vi "PMT communication_MD.vi"   [LabVIEW 2012]
uses:
  GFG/GFGstringGet.vi
  <vilib>/Instr/_visa.llb/VISA Configure Serial Port (Instr).vi
  GFG/GFGnumericGet.vi
  GFG/GFG library.lvlib
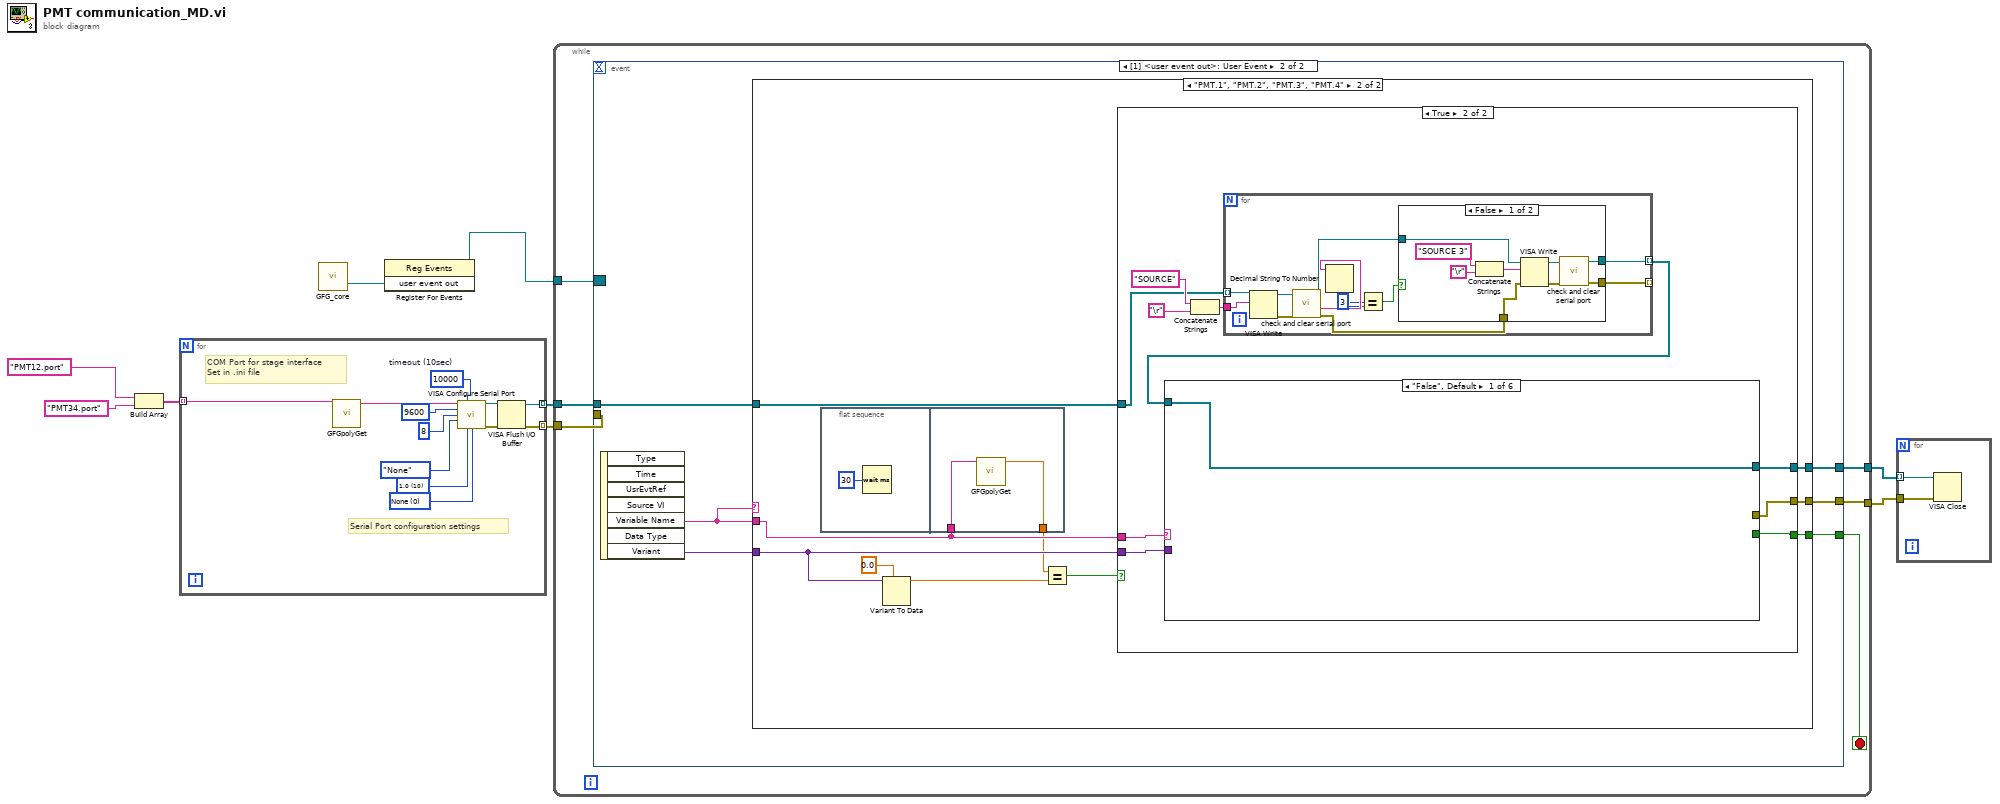
[diagram p0: block diagram]
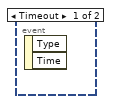
[diagram p2: hidden frame]
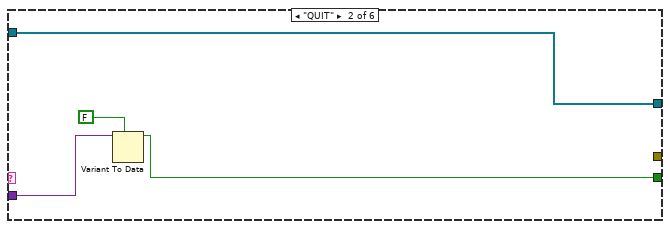
[diagram p6: hidden frame]
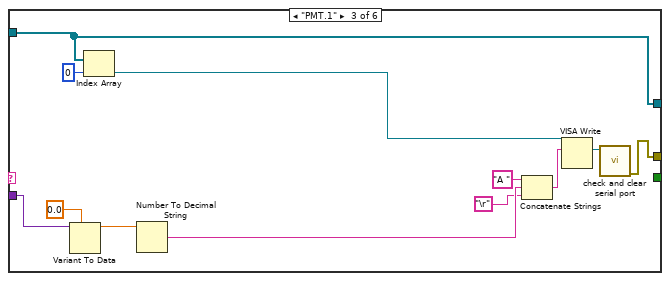
[diagram p7: hidden frame]
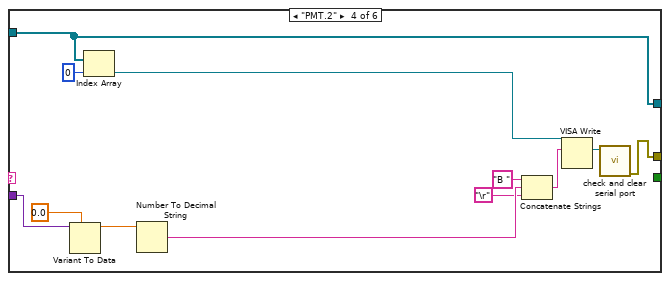
[diagram p8: hidden frame]
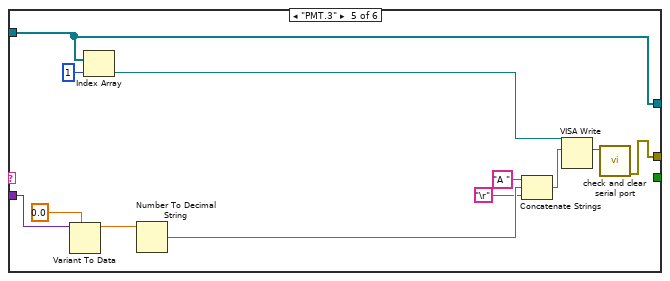
[diagram p9: hidden frame]
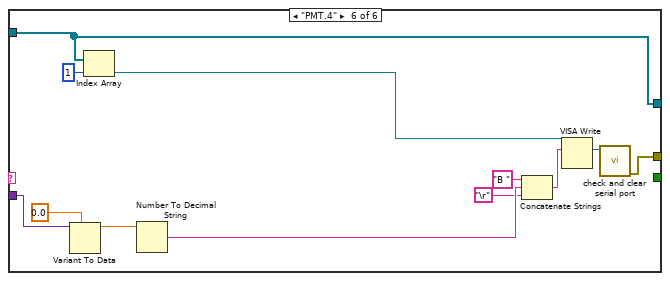
[diagram p10: hidden frame]
diagram:
  n1 = Build Array("PMT12.port" ("Variable Name in"), "PMT34.port" ("Variable Name in")) -> (w1:string[])
  n2 = for {
    tunnel: [w12] -> w9 mode=indexing
    tunnel: [w11] -> w8 mode=indexing
    tunnel: w1 -> [w10] mode=indexing
    w16 = u16 0 items=["None", "XON/XOFF", "RTS/CTS", "XON/XOFF & RTS/CTS", "DTR/DSR", "XON/XOFF & DTR/DSR"] ("flow control (0:none)")
    w17 = u16 10 items=["1.0"=10, "1.5"=15, "2.0"=20] ("stop bits (10: 1 bit)")
    w21 = u32 10000  # timeout (10sec)
    # "COM Port for stage interface\nSet in .ini file"
    # "Serial Port configuration settings"
    n3 = call-poly "GFGpolyGet.vi"("Variable Name in"=w10) -> ("String"=w13:string)  [unwired: 10 in]
    n4 = call-poly "VISA Configure Serial Port"("VISA resource name"=w13, "timeout (10sec)"=w21, "baud rate (9600)"=u32 9600, "data bits (8)"=u16 8, "parity (0:none)"=enum16{"None", "Odd", "Even", "Mark", "Space"}."None", "stop bits (10: 1 bit)"=w17, "flow control (0:none)"=w16) -> ("VISA resource name out"=w15:refnum<visa-resource-name>, "error out"=w14:errorcluster)  [unwired: 7 in]
    n5 = VISA Flush I/O Buffer(VISA resource name=w15, error in (no error)=w14) -> (VISA resource name out=w11:refnum<visa-resource-name>, error out=w12:errorcluster)  [unwired: 1 in]
  }
  n6 = call "GFG_core.vi"() -> ("user event out"=w2:refnum<user-event>)  [unwired: 13 in, 6 out]
  n7 = register-events(w2) -> (reference out=w5:refnum<event-registration>)  [unwired: 2 in, 1 out]
  n8 = while {
    tunnel: [w27] -> w7
    tunnel: w8 -> [w26]
    tunnel: w9 -> [w24]
    tunnel: [w23] -> w6
    tunnel: w5 -> [w22]
    stop <- w25 stop-if-true
    n9 = event shown="[1] <user event out>: User Event" {
      selector: w22 -> [_ _]
      dyn-events: _ -> [_ _]
      timeout: _ -> [_ _]
      tunnel: [_ w30] -> w27
      tunnel: w26 -> [_ w31]
      tunnel: [_ w32] -> w25
      tunnel: w24 -> [_ _]
      tunnel: [_ w29] -> w23
      event Timeout {
        n10 = event-data() -> ()  [unwired: 1 in, 2 out]
      }
      event User Event {
        n11 = event-data() -> ("Variable Name"=w28:string, "Variant"=w33:variant)  [unwired: 1 in, 5 out]
        n12 = case shown="\"PMT.1\", \"PMT.2\", \"PMT.3\", \"PMT.4\"" w28 {
          tunnel: w28 -> [_ w38]
          tunnel: w33 -> [_ w40]
          tunnel: [_ w44] -> w32
          tunnel: w31 -> [w34 w43]
          tunnel: [w34 w42] -> w30
          tunnel: [_ w41] -> w29
          frame "False", Default {
          }
          frame "PMT.1", "PMT.2", "PMT.3", "PMT.4" {
            n13 = flat-sequence {
              tunnel: w38 -> [w47]
              tunnel: [w46] -> w37
              frame #0 {
                n14 = Wait (ms)(milliseconds to wait=u32 30) -> ()  [unwired: 1 out]
              }
              frame #1 {
                n15 = call-poly "GFGpolyGet.vi"("Variable Name in"=w47) -> ("Numeric"=w46:dbl)  [unwired: 9 in, 1 out]
              }
            }
            n16 = Variant To Data(type=0.0, Variant=w40) -> (data=w36:dbl)  [unwired: 1 in, 1 out]
            n17 = Equal?(x=w37, y=w36) -> (x = y?=w35:bool)
            n18 = case shown="True" w35 {
              tunnel: w38 -> [_ w58]
              tunnel: w40 -> [_ w57]
              tunnel: [_ w56] -> w44
              tunnel: w43 -> [w48 w50]
              tunnel: [w48 w55] -> w42
              tunnel: [_ w54] -> w41
              frame False {
              }
              frame True {
                n19 = Concatenate Strings("SOURCE" ("write buffer"), "\r") -> (w53:string)
                n20 = for {
                  tunnel: w53 -> [w70]
                  tunnel: w50 -> [w68] mode=indexing
                  tunnel: [w63] -> _ mode=indexing
                  tunnel: [w62] -> w49 mode=indexing
                  n21 = VISA Write(VISA resource name=w68, write buffer=w70) -> (VISA resource name out=w69:refnum<visa-resource-name>, error out=w67:errorcluster)  [unwired: 1 in, 1 out]
                  n22 = call "check and clear serial port.vi"("error in (no error)"=w67, "VISA resource name in"=w69) -> ("error out"=w64:errorcluster, "read buffer"=w61:string, "VISA resource name out"=w65:refnum<visa-resource-name>)  [unwired: 6 in, 1 out]
                  n23 = Decimal String To Number(string=w61) -> (number=w60:i32)  [unwired: 2 in, 1 out]
                  n24 = Equal?(x=3, y=w60) -> (x = y?=w66:bool)
                  n25 = case shown="False" w66 {
                    tunnel: w65 -> [w75 w80]
                    tunnel: w64 -> [w73 w81]
                    tunnel: [w72 w81] -> w63
                    tunnel: [w71 w80] -> w62
                    frame False {
                      n26 = Concatenate Strings("SOURCE 3" ("write buffer"), "\r") -> (w76:string)
                      n27 = VISA Write(VISA resource name=w75, write buffer=w76, error in (no error)=w73) -> (VISA resource name out=w79:refnum<visa-resource-name>, error out=w74:errorcluster)  [unwired: 1 out]
                      n28 = call "check and clear serial port.vi"("error in (no error)"=w74, "VISA resource name in"=w79) -> ("error out"=w72:errorcluster, "VISA resource name out"=w71:refnum<visa-resource-name>)  [unwired: 6 in, 2 out]
                    }
                    frame True {
                    }
                  }
                }
                n29 = case shown="\"False\", Default" w58 {
                  tunnel: [_ w84 _ _ _ _] -> w56
                  tunnel: w57 -> [_ w86 w96 w108 w120 w132]
                  tunnel: w49 -> [w82 w83 w97 w109 w121 w133]
                  tunnel: [w82 w83 w97 w109 w121 w133] -> w55
                  tunnel: [_ _ w92 w104 w116 w128] -> w54
                  frame "False", Default {
                  }
                  frame "QUIT" {
                    n30 = Variant To Data(type=FALSE ("NewVal"), Variant=w86) -> (data=w84:bool)  [unwired: 1 in, 1 out]
                  }
                  frame "PMT.1" {
                    n31 = Variant To Data(type=0.0, Variant=w96) -> (data=w94:dbl)  [unwired: 1 in, 1 out]
                    n32 = Index Array(array=w97, index=0) -> (element=w87:refnum<visa-resource-name>)
                    n33 = Number To Decimal String(number=w94) -> (decimal integer string=w93:string)  [unwired: 1 in]
                    n34 = Concatenate Strings("A " ("string"), w93, "\r") -> (w89:string)
                    n35 = VISA Write(VISA resource name=w87, write buffer=w89) -> (VISA resource name out=w91:refnum<visa-resource-name>)  [unwired: 1 in, 2 out]
                    n36 = call "check and clear serial port.vi"("VISA resource name in"=w91) -> ("error out"=w92:errorcluster)  [unwired: 7 in, 3 out]
                  }
                  frame "PMT.2" {
                    n37 = Variant To Data(type=0.0, Variant=w108) -> (data=w106:dbl)  [unwired: 1 in, 1 out]
                    n38 = Index Array(array=w109, index=0) -> (element=w99:refnum<visa-resource-name>)
                    n39 = Number To Decimal String(number=w106) -> (decimal integer string=w105:string)  [unwired: 1 in]
                    n40 = Concatenate Strings("B " ("string"), w105, "\r") -> (w101:string)
                    n41 = VISA Write(VISA resource name=w99, write buffer=w101) -> (VISA resource name out=w103:refnum<visa-resource-name>)  [unwired: 1 in, 2 out]
                    n42 = call "check and clear serial port.vi"("VISA resource name in"=w103) -> ("error out"=w104:errorcluster)  [unwired: 7 in, 3 out]
                  }
                  frame "PMT.3" {
                    n43 = Variant To Data(type=0.0, Variant=w120) -> (data=w118:dbl)  [unwired: 1 in, 1 out]
                    n44 = Index Array(array=w121, index=1) -> (element=w111:refnum<visa-resource-name>)
                    n45 = Number To Decimal String(number=w118) -> (decimal integer string=w117:string)  [unwired: 1 in]
                    n46 = Concatenate Strings("A " ("string"), w117, "\r") -> (w113:string)
                    n47 = VISA Write(VISA resource name=w111, write buffer=w113) -> (VISA resource name out=w115:refnum<visa-resource-name>)  [unwired: 1 in, 2 out]
                    n48 = call "check and clear serial port.vi"("VISA resource name in"=w115) -> ("error out"=w116:errorcluster)  [unwired: 7 in, 3 out]
                  }
                  frame "PMT.4" {
                    n49 = Variant To Data(type=0.0, Variant=w132) -> (data=w130:dbl)  [unwired: 1 in, 1 out]
                    n50 = Index Array(array=w133, index=1) -> (element=w123:refnum<visa-resource-name>)
                    n51 = Number To Decimal String(number=w130) -> (decimal integer string=w129:string)  [unwired: 1 in]
                    n52 = Concatenate Strings("B " ("string"), w129, "\r") -> (w125:string)
                    n53 = VISA Write(VISA resource name=w123, write buffer=w125) -> (VISA resource name out=w127:refnum<visa-resource-name>)  [unwired: 1 in, 2 out]
                    n54 = call "check and clear serial port.vi"("VISA resource name in"=w127) -> ("error out"=w128:errorcluster)  [unwired: 7 in, 3 out]
                  }
                }
              }
            }
          }
        }
      }
    }
  }
  n55 = for {
    tunnel: w7 -> [w136] mode=indexing
    tunnel: w6 -> [w135]
    n56 = VISA Close(VISA resource name=w136, error in (no error)=w135) -> ()  [unwired: 1 out]
  }
